vi "test-pose2d.vi"(8 "error in (no error)":errorcluster) -> (0 "error out":errorcluster, 3 "All PASSED":bool)   [LabVIEW 2019]
uses:
  <vilib>/Rock Robotics/WPI/ThirdParty/JAS_Junk/TrajLib/Rotation2d_GetAngleCosSin.vi
  <vilib>/Rock Robotics/WPI/ThirdParty/JAS_Junk/TrajLib/Translation2d_GetDistance.vi
  <vilib>/Rock Robotics/WPI/ThirdParty/JAS_Junk/TrajLib/Rotation2d_Minus.vi
  <vilib>/Rock Robotics/WPI/ThirdParty/JAS_Junk/TrajLib/Translation2d_Equals.vi
  <vilib>/Rock Robotics/WPI/ThirdParty/JAS_Junk/TrajLib/Rotation2d_Equals.vi
  <vilib>/Rock Robotics/WPI/ThirdParty/JAS_Junk/TrajLib/Transform2d_Create_PosePose.vi
  <vilib>/Rock Robotics/WPI/ThirdParty/JAS_Junk/TrajLib/Pose2d_TransformBy.vi
  <vilib>/Rock Robotics/WPI/ThirdParty/JAS_Junk/TrajLib/Util_CalcDist.vi
  <vilib>/Rock Robotics/WPI/ThirdParty/JAS_Junk/TrajLib/Rotation2d_UnaryMinus.vi
  <vilib>/Rock Robotics/WPI/ThirdParty/JAS_Junk/TrajLib/Rotation2d_RotateBy.vi
  <vilib>/Rock Robotics/WPI/ThirdParty/JAS_Junk/TrajLib/Translation2d_RotateBy.vi
  <vilib>/Rock Robotics/WPI/ThirdParty/JAS_Junk/TrajLib/Translation2d_Minus.vi
  <vilib>/Rock Robotics/WPI/ThirdParty/JAS_Junk/TrajLib/Translation2d_Plus.vi
  <vilib>/Rock Robotics/WPI/ThirdParty/JAS_Junk/TrajLib/Rotation2d_Plus.vi
  <vilib>/Rock Robotics/WPI/ThirdParty/JAS_Junk/TrajLib/Rotation2d_CreateXY.vi
  <vilib>/Rock Robotics/WPI/ThirdParty/JAS_Junk/TrajLib/Trajectory_Library.lvlib
panel:
  out "Nearest To":bool
  out "T4 -- Deg -- 0":dbl
  out "T4 -- y -- 0":dbl
  out "T4 -- X -- 0":dbl
  out "T3 - False":bool
  out "T2 - True":bool
  out "T1 -- Deg -- 0":dbl
  out "T1 -- y -- 0":dbl
  out "T1 -- X -- 0":dbl
  out "T0 -- Deg -- 0":dbl
  out "T0 -- y -- 0":dbl
  out "T0 -- X -- 0":dbl
  # "Pose 2D test"
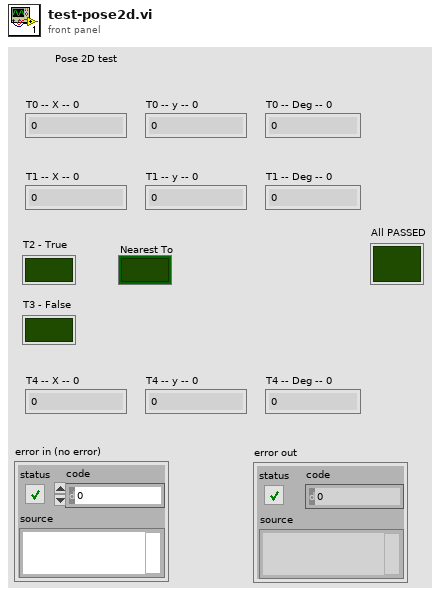
[diagram p1: front panel]
types:
  T1 = typedef "Trajectory_Library.lvlib/TRANSLATION2D.ctl" = cluster{"X":dbl, "Y":dbl}
  T2 = typedef "Trajectory_Library.lvlib/ROTATION2D.ctl" = cluster{"VALUE":dbl, "COS":dbl, "SIN":dbl}
  T3 = typedef "Trajectory_Library.lvlib/POSE2D.ctl" = cluster{"TRANSLATION":T1, "ROTATION":T2}
  T4 = typedef "Trajectory_Library.lvlib/TRANSFORM2D.ctl" = cluster{"TRANSLATION":T1, "ROTATION":T2, "xF":bool}
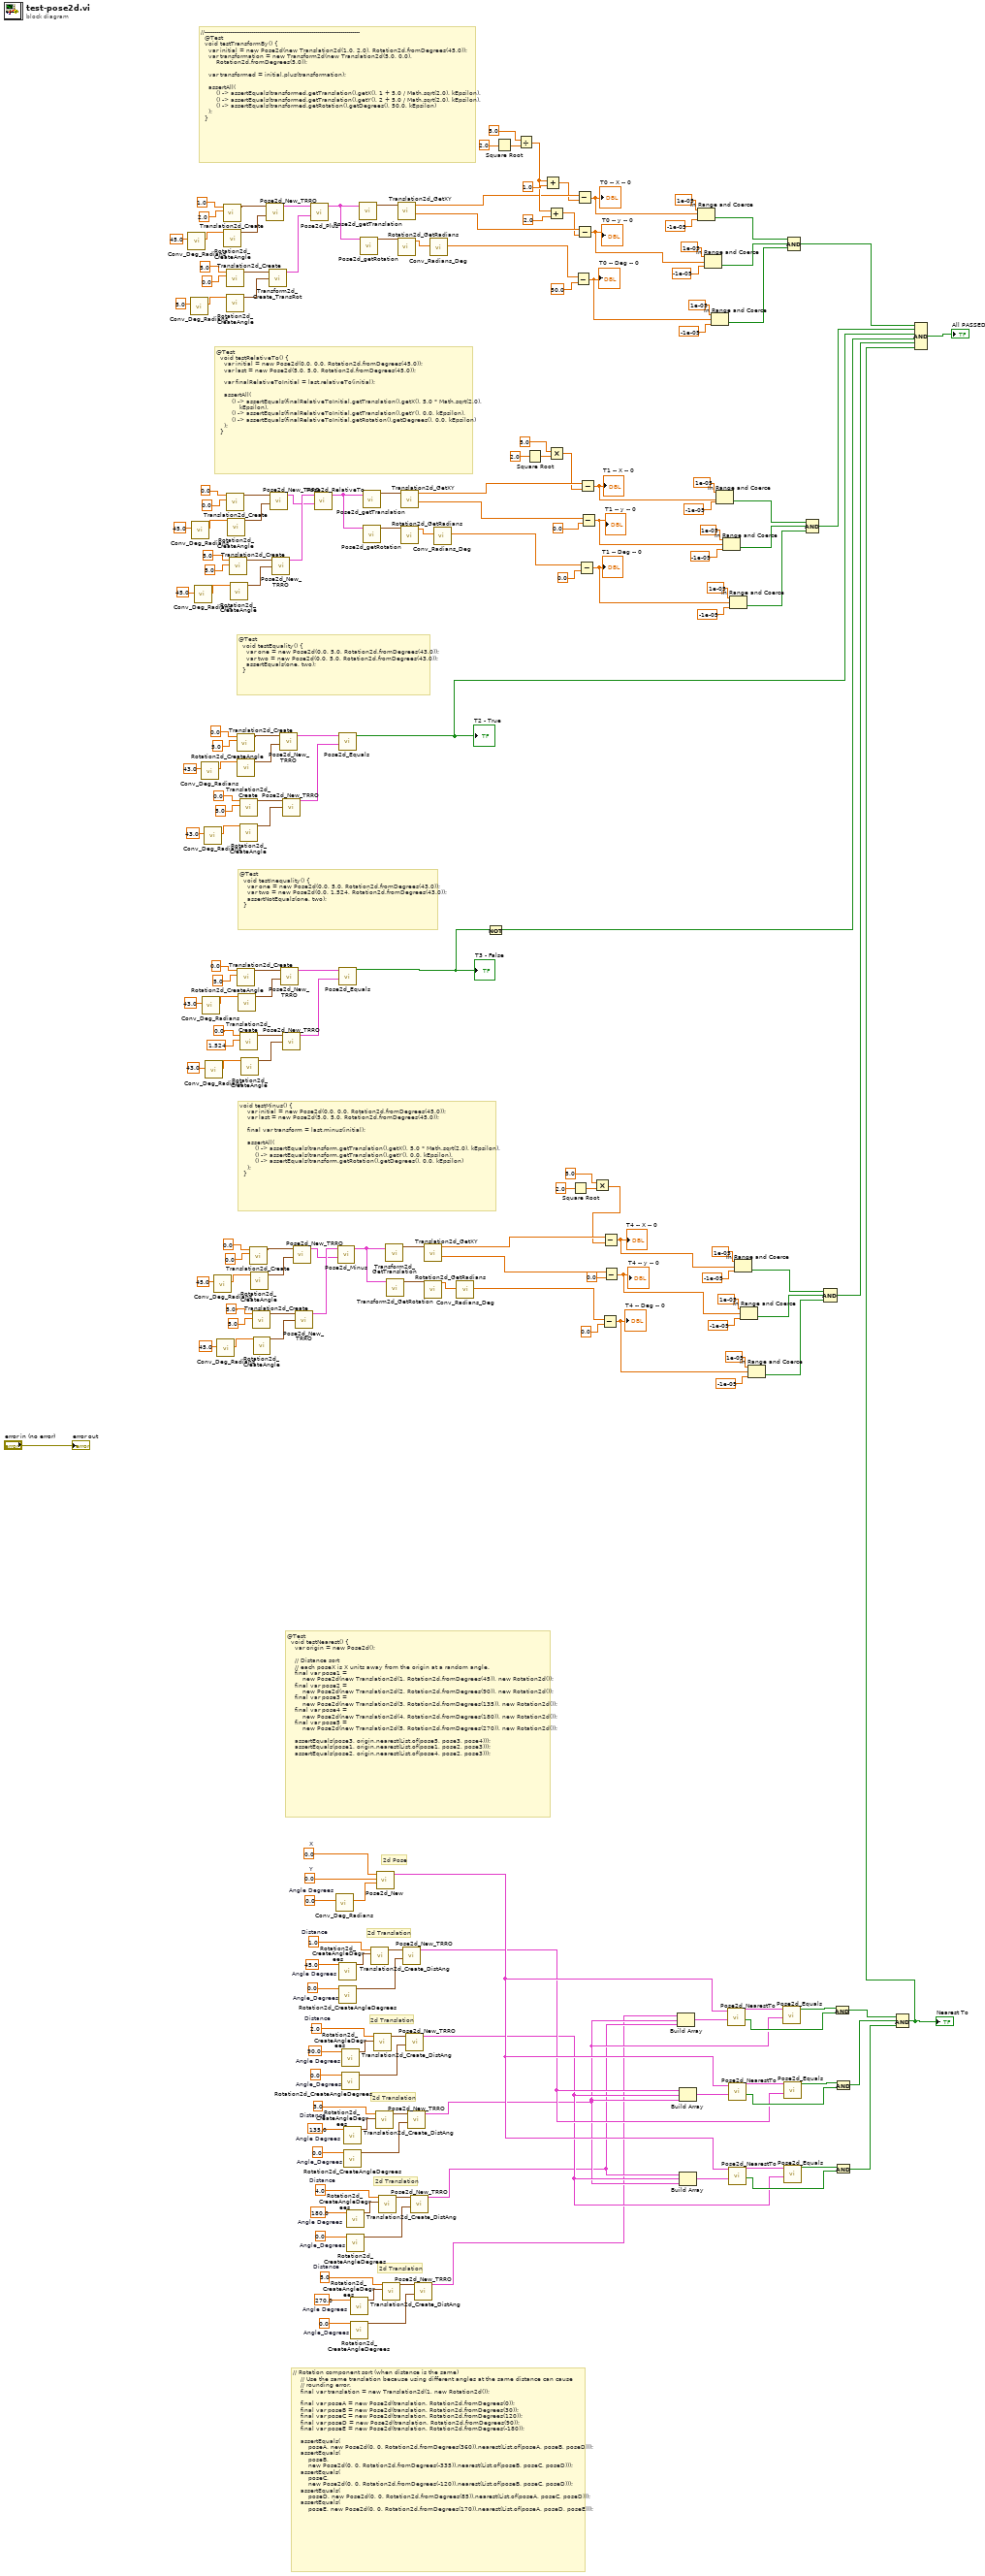
[diagram p0: block diagram]
diagram:
  w5 = 0.0  # Angle_Degrees
  w6 = 5.0  # Distance
  w8 = 270.0  # Angle Degrees
  w12 = 0.0  # Angle_Degrees
  w13 = 4.0  # Distance
  w15 = 180.0  # Angle Degrees
  w19 = 0.0  # Angle_Degrees
  w20 = 3.0  # Distance
  w22 = 135.0  # Angle Degrees
  w26 = 0.0  # Angle_Degrees
  w27 = 2.0  # Distance
  w29 = 90.0  # Angle Degrees
  w33 = 0.0  # Angle_Degrees
  w50 = 1.0  # Distance
  w52 = 45.0  # Angle Degrees
  w56 = 0.0  # X
  w55 = 0.0  # Y
  w53 = 0.0  # Angle Degrees
  # "// Rotation component sort (when distance is the same)\n    // Use the same translation because using different angles at the same distance can cause\n    // rounding error.\n    final var translation = new Translation2d(1, new Rotation2d());\n\n    final var poseA = new Pose2d(translation, Rotation2d.fromDegrees(0));\n    final var poseB = new Pose2d(translation, Rotation2d.fromDegrees(30));\n    final var poseC = new Pose2d(translation, Rotation2d.fromDegrees(120));\n    final var poseD = new Pose2d(translation, Rotation2d.fromDegrees(90));\n    final var poseE = new Pose2d(translation, Rotation2d.fromDegrees(-180));\n\n    assertEquals(\n        poseA, new Pose2d(0, 0, Rotation2d.fromDegrees(360)).nearest(List.of(poseA, poseB, poseD)));\n    assertEquals(\n        poseB,\n        new Pose2d(0, 0, Rotation2d.fromDegrees(-335)).nearest(List.of(poseB, poseC, poseD)));\n    assertEquals(\n        poseC,\n        new Pose2d(0, 0, Rotation2d.fromDegrees(-120)).nearest(List.of(poseB, poseC, poseD)));\n    assertEquals(\n        poseD, new Pose2d(0, 0, Rotation2d.fromDegrees(85)).nearest(List.of(poseA, poseC, poseD)));\n    assertEquals(\n        poseE, new Pose2d(0, 0, Rotation2d.fromDegrees(170)).nearest(List.of(poseA, poseD, poseE)));"
  # "2d Translation"
  # "2d Translation"
  # "2d Translation"
  # "2d Translation"
  # "2d Translation"
  # "2d Pose"
  # "@Test\n  void testNearest() {\n    var origin = new Pose2d();\n\n    // Distance sort\n    // each poseX is X units away from the origin at a random angle.\n    final var pose1 =\n        new Pose2d(new Translation2d(1, Rotation2d.fromDegrees(45)), new Rotation2d());\n    final var pose2 =\n        new Pose2d(new Translation2d(2, Rotation2d.fromDegrees(90)), new Rotation2d());\n    final var pose3 =\n        new Pose2d(new Translation2d(3, Rotation2d.fromDegrees(135)), new Rotation2d());\n    final var pose4 =\n        new Pose2d(new Translation2d(4, Rotation2d.fromDegrees(180)), new Rotation2d());\n    final var pose5 =\n        new Pose2d(new Translation2d(5, Rotation2d.fromDegrees(270)), new Rotation2d());\n\n    assertEquals(pose3, origin.nearest(List.of(pose5, pose3, pose4)));\n    assertEquals(pose1, origin.nearest(List.of(pose1, pose2, pose3)));\n    assertEquals(pose2, origin.nearest(List.of(pose4, pose2, pose3)));"
  # "//--------------------------------------------------------------------------------\n  @Test\n  void testTransformBy() {\n    var initial = new Pose2d(new Translation2d(1.0, 2.0), Rotation2d.fromDegrees(45.0));\n    var transformation = new Transform2d(new Translation2d(5.0, 0.0),\n        Rotation2d.fromDegrees(5.0));\n\n    var transformed = initial.plus(transformation);\n\n    assertAll(\n        () -> assertEquals(transformed.getTranslation().getX(), 1 + 5.0 / Math.sqrt(2.0), kEpsilon),\n        () -> assertEquals(transformed.getTranslation().getY(), 2 + 5.0 / Math.sqrt(2.0), kEpsilon),\n        () -> assertEquals(transformed.getRotation().getDegrees(), 50.0, kEpsilon)\n    );\n  }"
  # "void testMinus() {\n    var initial = new Pose2d(0.0, 0.0, Rotation2d.fromDegrees(45.0));\n    var last = new Pose2d(5.0, 5.0, Rotation2d.fromDegrees(45.0));\n\n    final var transform = last.minus(initial);\n\n    assertAll(\n        () -> assertEquals(transform.getTranslation().getX(), 5.0 * Math.sqrt(2.0), kEpsilon),\n        () -> assertEquals(transform.getTranslation().getY(), 0.0, kEpsilon),\n        () -> assertEquals(transform.getRotation().getDegrees(), 0.0, kEpsilon)\n    );\n  }"
  # "@Test\n  void testInequality() {\n    var one = new Pose2d(0.0, 5.0, Rotation2d.fromDegrees(43.0));\n    var two = new Pose2d(0.0, 1.524, Rotation2d.fromDegrees(43.0));\n    assertNotEquals(one, two);\n  }"
  # "@Test\n  void testEquality() {\n    var one = new Pose2d(0.0, 5.0, Rotation2d.fromDegrees(43.0));\n    var two = new Pose2d(0.0, 5.0, Rotation2d.fromDegrees(43.0));\n    assertEquals(one, two);\n  }"
  # "@Test\n  void testRelativeTo() {\n    var initial = new Pose2d(0.0, 0.0, Rotation2d.fromDegrees(45.0));\n    var last = new Pose2d(5.0, 5.0, Rotation2d.fromDegrees(45.0));\n\n    var finalRelativeToInitial = last.relativeTo(initial);\n\n    assertAll(\n        () -> assertEquals(finalRelativeToInitial.getTranslation().getX(), 5.0 * Math.sqrt(2.0),\n            kEpsilon),\n        () -> assertEquals(finalRelativeToInitial.getTranslation().getY(), 0.0, kEpsilon),\n        () -> assertEquals(finalRelativeToInitial.getRotation().getDegrees(), 0.0, kEpsilon)\n    );\n  }"
  n1 = call <vilib>:"Conv_Deg_Radians.vi"("Degress"=45.0) -> ("Radians"=w209:dbl)  [unwired: 10 in]
  n2 = call <vilib>:"Conv_Deg_Radians.vi"("Degress"=5.0) -> ("Radians"=w204:dbl)  [unwired: 10 in]
  n3 = call <vilib>:"Conv_Deg_Radians.vi"("Degress"=45.0) -> ("Radians"=w179:dbl)  [unwired: 10 in]
  n4 = call <vilib>:"Conv_Deg_Radians.vi"("Degress"=45.0) -> ("Radians"=w174:dbl)  [unwired: 10 in]
  n5 = call <vilib>:"Conv_Deg_Radians.vi"("Degress"=43.0) -> ("Radians"=w152:dbl)  [unwired: 10 in]
  n6 = call <vilib>:"Conv_Deg_Radians.vi"("Degress"=43.0) -> ("Radians"=w138:dbl)  [unwired: 10 in]
  n7 = call <vilib>:"Conv_Deg_Radians.vi"("Degress"=43.0) -> ("Radians"=w147:dbl)  [unwired: 10 in]
  n8 = call <vilib>:"Conv_Deg_Radians.vi"("Degress"=43.0) -> ("Radians"=w133:dbl)  [unwired: 10 in]
  n9 = call <vilib>:"Conv_Deg_Radians.vi"("Degress"=45.0) -> ("Radians"=w124:dbl)  [unwired: 10 in]
  n10 = call <vilib>:"Conv_Deg_Radians.vi"("Degress"=45.0) -> ("Radians"=w119:dbl)  [unwired: 10 in]
  n11 = call <vilib>:"Translation2d_Create.vi"("Y"=2.0, "X"=1.0) -> ("TRANSLATION"=w208:T1)  [unwired: 9 in]
  n12 = call <vilib>:"Rotation2d_CreateAngle.vi"("Angle"=w209) -> ("ROTATION"=w207:T2)  [unwired: 10 in]
  n13 = call <vilib>:"Translation2d_Create.vi"("Y"=0.0, "X"=5.0) -> ("TRANSLATION"=w202:T1)  [unwired: 9 in]
  n14 = call <vilib>:"Rotation2d_CreateAngle.vi"("Angle"=w204) -> ("ROTATION"=w201:T2)  [unwired: 10 in]
  n15 = call <vilib>:"Translation2d_Create.vi"("Y"=0.0, "X"=0.0) -> ("TRANSLATION"=w178:T1)  [unwired: 9 in]
  n16 = call <vilib>:"Rotation2d_CreateAngle.vi"("Angle"=w179) -> ("ROTATION"=w177:T2)  [unwired: 10 in]
  n17 = call <vilib>:"Translation2d_Create.vi"("Y"=5.0, "X"=5.0) -> ("TRANSLATION"=w172:T1)  [unwired: 9 in]
  n18 = call <vilib>:"Rotation2d_CreateAngle.vi"("Angle"=w174) -> ("ROTATION"=w171:T2)  [unwired: 10 in]
  n19 = call <vilib>:"Translation2d_Create.vi"("Y"=5.0, "X"=0.0) -> ("TRANSLATION"=w151:T1)  [unwired: 9 in]
  n20 = call <vilib>:"Rotation2d_CreateAngle.vi"("Angle"=w152) -> ("ROTATION"=w150:T2)  [unwired: 10 in]
  n21 = call <vilib>:"Translation2d_Create.vi"("Y"=5.0, "X"=0.0) -> ("TRANSLATION"=w137:T1)  [unwired: 9 in]
  n22 = call <vilib>:"Rotation2d_CreateAngle.vi"("Angle"=w138) -> ("ROTATION"=w136:T2)  [unwired: 10 in]
  n23 = call <vilib>:"Translation2d_Create.vi"("Y"=5.0, "X"=0.0) -> ("TRANSLATION"=w145:T1)  [unwired: 9 in]
  n24 = call <vilib>:"Rotation2d_CreateAngle.vi"("Angle"=w147) -> ("ROTATION"=w144:T2)  [unwired: 10 in]
  n25 = call <vilib>:"Translation2d_Create.vi"("Y"=1.524, "X"=0.0) -> ("TRANSLATION"=w131:T1)  [unwired: 9 in]
  n26 = call <vilib>:"Rotation2d_CreateAngle.vi"("Angle"=w133) -> ("ROTATION"=w130:T2)  [unwired: 10 in]
  n27 = call <vilib>:"Translation2d_Create.vi"("Y"=0.0, "X"=0.0) -> ("TRANSLATION"=w123:T1)  [unwired: 9 in]
  n28 = call <vilib>:"Rotation2d_CreateAngle.vi"("Angle"=w124) -> ("ROTATION"=w122:T2)  [unwired: 10 in]
  n29 = call <vilib>:"Translation2d_Create.vi"("Y"=5.0, "X"=5.0) -> ("TRANSLATION"=w117:T1)  [unwired: 9 in]
  n30 = call <vilib>:"Rotation2d_CreateAngle.vi"("Angle"=w119) -> ("ROTATION"=w116:T2)  [unwired: 10 in]
  n31 = call <vilib>:"Pose2d_New_TRRO.vi"("ROTATION"=w207, "TRANSLATION"=w208) -> ("outPOSE"=w200:T3)  [unwired: 9 in]
  n32 = call <vilib>:"Transform2d_Create_TransRot.vi"("ROTATION"=w201, "TRANSLATION"=w202) -> ("TRANSFORM"=w199:T4)  [unwired: 9 in]
  n33 = call <vilib>:"Pose2d_New_TRRO.vi"("ROTATION"=w177, "TRANSLATION"=w178) -> ("outPOSE"=w157:T3)  [unwired: 9 in]
  n34 = call <vilib>:"Pose2d_New_TRRO.vi"("ROTATION"=w171, "TRANSLATION"=w172) -> ("outPOSE"=w158:T3)  [unwired: 9 in]
  n35 = call <vilib>:"Pose2d_New_TRRO.vi"("ROTATION"=w150, "TRANSLATION"=w151) -> ("outPOSE"=w143:T3)  [unwired: 9 in]
  n36 = call <vilib>:"Pose2d_New_TRRO.vi"("ROTATION"=w136, "TRANSLATION"=w137) -> ("outPOSE"=w129:T3)  [unwired: 9 in]
  n37 = call <vilib>:"Pose2d_New_TRRO.vi"("ROTATION"=w144, "TRANSLATION"=w145) -> ("outPOSE"=w142:T3)  [unwired: 9 in]
  n38 = call <vilib>:"Pose2d_New_TRRO.vi"("ROTATION"=w130, "TRANSLATION"=w131) -> ("outPOSE"=w128:T3)  [unwired: 9 in]
  n39 = call <vilib>:"Pose2d_New_TRRO.vi"("ROTATION"=w122, "TRANSLATION"=w123) -> ("outPOSE"=w103:T3)  [unwired: 9 in]
  n40 = call <vilib>:"Pose2d_New_TRRO.vi"("ROTATION"=w116, "TRANSLATION"=w117) -> ("outPOSE"=w104:T3)  [unwired: 9 in]
  n41 = call <vilib>:"Pose2d_Plus.vi"("other TRANSFORM"=w199, "in POSE"=w200) -> ("out POSE"=w197:T3)  [unwired: 9 in]
  n42 = call <vilib>:"Pose2d_RelativeTo.vi"("other POSE"=w157, "in POSE"=w158) -> ("out POSE"=w169:T3)  [unwired: 9 in]
  n43 = call <vilib>:"Conv_Deg_Radians.vi"("Degress"=w53) -> ("Radians"=w54:dbl)  [unwired: 10 in]
  n44 = call <vilib>:"Pose2d_Minus.vi"("other POSE"=w103, "in POSE"=w104) -> ("outTRANSFORM"=w114:T4)  [unwired: 9 in]
  n45 = call <vilib>:"Pose2d_Equals.vi"("other POSE"=w142, "in POSE"=w143) -> ("Equals"=w73:bool)  [unwired: 9 in]
  "T2 - True" <- w73
  n46 = call <vilib>:"Pose2d_Equals.vi"("other POSE"=w128, "in POSE"=w129) -> ("Equals"=w72:bool)  [unwired: 9 in]
  "T3 - False" <- w72
  n47 = call <vilib>:"Rotation2d_CreateAngleDegrees.vi"("Angle_Degrees"=w52) -> ("ROTATION"=w51:T2)  [unwired: 10 in]
  n48 = call <vilib>:"Rotation2d_CreateAngleDegrees.vi"("Angle_Degrees"=w33) -> ("ROTATION"=w31:T2)  [unwired: 10 in]
  n49 = call <vilib>:"Rotation2d_CreateAngleDegrees.vi"("Angle_Degrees"=w29) -> ("ROTATION"=w28:T2)  [unwired: 10 in]
  n50 = call <vilib>:"Rotation2d_CreateAngleDegrees.vi"("Angle_Degrees"=w26) -> ("ROTATION"=w24:T2)  [unwired: 10 in]
  n51 = call <vilib>:"Rotation2d_CreateAngleDegrees.vi"("Angle_Degrees"=w22) -> ("ROTATION"=w21:T2)  [unwired: 10 in]
  n52 = call <vilib>:"Rotation2d_CreateAngleDegrees.vi"("Angle_Degrees"=w19) -> ("ROTATION"=w17:T2)  [unwired: 10 in]
  n53 = call <vilib>:"Rotation2d_CreateAngleDegrees.vi"("Angle_Degrees"=w15) -> ("ROTATION"=w14:T2)  [unwired: 10 in]
  n54 = call <vilib>:"Rotation2d_CreateAngleDegrees.vi"("Angle_Degrees"=w12) -> ("ROTATION"=w10:T2)  [unwired: 10 in]
  n55 = call <vilib>:"Rotation2d_CreateAngleDegrees.vi"("Angle_Degrees"=w8) -> ("ROTATION"=w7:T2)  [unwired: 10 in]
  n56 = call <vilib>:"Rotation2d_CreateAngleDegrees.vi"("Angle_Degrees"=w5) -> ("ROTATION"=w3:T2)  [unwired: 10 in]
  n57 = call <vilib>:"Pose2d_getTranslation.vi"("in POSE"=w197) -> ("outTRANSLATION"=w198:T1)  [unwired: 10 in]
  n58 = call <vilib>:"Pose2d_getRotation.vi"("in POSE"=w197) -> ("out ROTATION"=w196:T2)  [unwired: 10 in]
  n59 = call <vilib>:"Pose2d_getTranslation.vi"("in POSE"=w169) -> ("outTRANSLATION"=w170:T1)  [unwired: 10 in]
  n60 = call <vilib>:"Pose2d_getRotation.vi"("in POSE"=w169) -> ("out ROTATION"=w168:T2)  [unwired: 10 in]
  n61 = call <vilib>:"Translation2d_Create_DistAng.vi"("Angle"=w51, "Dist"=w50) -> ("TRANSLATION"=w32:T1)  [unwired: 9 in]
  n62 = call <vilib>:"Translation2d_Create_DistAng.vi"("Angle"=w28, "Dist"=w27) -> ("TRANSLATION"=w25:T1)  [unwired: 9 in]
  n63 = call <vilib>:"Translation2d_Create_DistAng.vi"("Angle"=w21, "Dist"=w20) -> ("TRANSLATION"=w18:T1)  [unwired: 9 in]
  n64 = call <vilib>:"Pose2d_New.vi"("Heading"=w54, "Y"=w55, "X"=w56) -> ("out POSe"=w34:T3)  [unwired: 8 in]
  n65 = call <vilib>:"Translation2d_Create_DistAng.vi"("Angle"=w14, "Dist"=w13) -> ("TRANSLATION"=w11:T1)  [unwired: 9 in]
  n66 = call <vilib>:"Translation2d_Create_DistAng.vi"("Angle"=w7, "Dist"=w6) -> ("TRANSLATION"=w4:T1)  [unwired: 9 in]
  n67 = call <vilib>:"Transform2d_GetTranslation.vi"("inTRANSFORM"=w114) -> ("TRANSLATION"=w115:T1)  [unwired: 10 in]
  n68 = call <vilib>:"Transform2d_GetRotation.vi"("inTRANSFORM"=w114) -> ("ROTATION"=w113:T2)  [unwired: 10 in]
  n69 = call <vilib>:"Translation2d_GetXY.vi"("In Translation"=w198) -> ("Y"=w187:dbl, "X"=w188:dbl)  [unwired: 9 in]
  n70 = call <vilib>:"Rotation2d_GetRadians.vi"("in ROTATION"=w196) -> ("AngleRadians"=w195:dbl)  [unwired: 10 in]
  n71 = call <vilib>:"Translation2d_GetXY.vi"("In Translation"=w170) -> ("Y"=w162:dbl, "X"=w163:dbl)  [unwired: 9 in]
  n72 = call <vilib>:"Rotation2d_GetRadians.vi"("in ROTATION"=w168) -> ("AngleRadians"=w167:dbl)  [unwired: 10 in]
  n73 = call <vilib>:"Pose2d_New_TRRO.vi"("ROTATION"=w31, "TRANSLATION"=w32) -> ("outPOSE"=w30:T3)  [unwired: 9 in]
  n74 = call <vilib>:"Pose2d_New_TRRO.vi"("ROTATION"=w24, "TRANSLATION"=w25) -> ("outPOSE"=w23:T3)  [unwired: 9 in]
  n75 = call <vilib>:"Pose2d_New_TRRO.vi"("ROTATION"=w17, "TRANSLATION"=w18) -> ("outPOSE"=w16:T3)  [unwired: 9 in]
  n76 = call <vilib>:"Pose2d_New_TRRO.vi"("ROTATION"=w10, "TRANSLATION"=w11) -> ("outPOSE"=w9:T3)  [unwired: 9 in]
  n77 = call <vilib>:"Pose2d_New_TRRO.vi"("ROTATION"=w3, "TRANSLATION"=w4) -> ("outPOSE"=w2:T3)  [unwired: 9 in]
  n78 = call <vilib>:"Translation2d_GetXY.vi"("In Translation"=w115) -> ("Y"=w107:dbl, "X"=w108:dbl)  [unwired: 9 in]
  n79 = call <vilib>:"Rotation2d_GetRadians.vi"("in ROTATION"=w113) -> ("AngleRadians"=w112:dbl)  [unwired: 10 in]
  n80 = call <vilib>:"Conv_Radians_Deg.vi"("Radians"=w195) -> ("Degrees"=w183:dbl)  [unwired: 10 in]
  n81 = call <vilib>:"Conv_Radians_Deg.vi"("Radians"=w167) -> ("Degrees"=w160:dbl)  [unwired: 10 in]
  n82 = call <vilib>:"Conv_Radians_Deg.vi"("Radians"=w112) -> ("Degrees"=w105:dbl)  [unwired: 10 in]
  n83 = Not(x=w72) -> (.not. x?=w71:bool)
  n84 = Square Root(x=2.0) -> (sqrt(x)=w193:dbl)
  n85 = Divide(x=5.0, y=w193) -> (x/y=w189:dbl)
  n86 = Square Root(x=2.0) -> (sqrt(x)=w165:dbl)
  n87 = Add(x=w189, y=1.0) -> (x+y=w185:dbl)
  n88 = Add(x=w189, y=2.0) -> (x+y=w186:dbl)
  n89 = Multiply(x=5.0, y=w165) -> (x*y=w156:dbl)
  n90 = Square Root(x=2.0) -> (sqrt(x)=w110:dbl)
  n91 = Subtract(x=w183, y=50.0) -> (x-y=w92:dbl)
  "T0 -- Deg -- 0" <- w92
  n92 = Subtract(x=w188, y=w185) -> (x-y=w94:dbl)
  "T0 -- X -- 0" <- w94
  n93 = Subtract(x=w187, y=w186) -> (x-y=w93:dbl)
  "T0 -- y -- 0" <- w93
  n94 = Subtract(x=w160, y=0.0) -> (x-y=w75:dbl)
  "T1 -- Deg -- 0" <- w75
  n95 = Subtract(x=w163, y=w156) -> (x-y=w77:dbl)
  "T1 -- X -- 0" <- w77
  n96 = Subtract(x=w162, y=0.0) -> (x-y=w76:dbl)
  "T1 -- y -- 0" <- w76
  n97 = Multiply(x=5.0, y=w110) -> (x*y=w102:dbl)
  n98 = Subtract(x=w105, y=0.0) -> (x-y=w59:dbl)
  "T4 -- Deg -- 0" <- w59
  n99 = Subtract(x=w108, y=w102) -> (x-y=w61:dbl)
  "T4 -- X -- 0" <- w61
  n100 = Subtract(x=w107, y=0.0) -> (x-y=w60:dbl)
  "T4 -- y -- 0" <- w60
  n101 = Build Array(w2, w16, w9) -> (w49:T3[])
  n102 = Build Array(w30, w23, w16) -> (w44:T3[])
  n103 = Build Array(w9, w23, w16) -> (w40:T3[])
  n104 = In Range and Coerce(upper limit=1e-05, x=w94, lower limit=-1e-05) -> (In Range?=w91:bool)  [unwired: 1 out]
  n105 = In Range and Coerce(upper limit=1e-05, x=w93, lower limit=-1e-05) -> (In Range?=w90:bool)  [unwired: 1 out]
  n106 = In Range and Coerce(upper limit=1e-05, x=w92, lower limit=-1e-05) -> (In Range?=w89:bool)  [unwired: 1 out]
  n107 = In Range and Coerce(upper limit=1e-05, x=w77, lower limit=-1e-05) -> (In Range?=w80:bool)  [unwired: 1 out]
  n108 = In Range and Coerce(upper limit=1e-05, x=w76, lower limit=-1e-05) -> (In Range?=w79:bool)  [unwired: 1 out]
  n109 = call <vilib>:"Pose2d_NearestTo.vi"("other POSE"=w49, "in POSE"=w34) -> ("Found"=w47:bool, "Nearest Pose"=w48:T3)  [unwired: 8 in]
  n110 = call <vilib>:"Pose2d_NearestTo.vi"("other POSE"=w44, "in POSE"=w34) -> ("Found"=w42:bool, "Nearest Pose"=w43:T3)  [unwired: 8 in]
  n111 = call <vilib>:"Pose2d_NearestTo.vi"("other POSE"=w40, "in POSE"=w34) -> ("Found"=w38:bool, "Nearest Pose"=w39:T3)  [unwired: 8 in]
  n112 = In Range and Coerce(upper limit=1e-05, x=w75, lower limit=-1e-05) -> (In Range?=w78:bool)  [unwired: 1 out]
  n113 = In Range and Coerce(upper limit=1e-05, x=w61, lower limit=-1e-05) -> (In Range?=w64:bool)  [unwired: 1 out]
  n114 = In Range and Coerce(upper limit=1e-05, x=w60, lower limit=-1e-05) -> (In Range?=w63:bool)  [unwired: 1 out]
  n115 = In Range and Coerce(upper limit=1e-05, x=w59, lower limit=-1e-05) -> (In Range?=w62:bool)  [unwired: 1 out]
  n116 = call <vilib>:"Pose2d_Equals.vi"("other POSE"=w16, "in POSE"=w48) -> ("Equals"=w46:bool)  [unwired: 9 in]
  n117 = call <vilib>:"Pose2d_Equals.vi"("other POSE"=w30, "in POSE"=w43) -> ("Equals"=w41:bool)  [unwired: 9 in]
  n118 = call <vilib>:"Pose2d_Equals.vi"("other POSE"=w23, "in POSE"=w39) -> ("Equals"=w37:bool)  [unwired: 9 in]
  n119 = Compound Arithmetic op=AND(w91, w90, w89) -> (w88:bool)
  n120 = Compound Arithmetic op=AND(w80, w79, w78) -> (w74:bool)
  n121 = Compound Arithmetic op=AND(w64, w63, w62) -> (w58:bool)
  n122 = And(x=w46, y=w47) -> (x .and. y?=w45:bool)
  n123 = And(x=w41, y=w42) -> (x .and. y?=w36:bool)
  n124 = And(x=w37, y=w38) -> (x .and. y?=w35:bool)
  n125 = Compound Arithmetic op=AND(w45, w36, w35) -> (w1:bool)
  "Nearest To" <- w1
  n126 = Compound Arithmetic op=AND(w88, w74, w73, w71, w58, w1) -> (→"All PASSED":bool)
  "error out" <- "error in (no error)"
